vi "Log Text to Sinks.vi"(8 "error in (no error)":errorcluster, 10 "Log Text":string, 11 "Logger in":refnum<class "Logger.lvclass">) -> (0 "error out":errorcluster, 3 "Logger out":refnum<class "Logger.lvclass">)   [LabVIEW 2020, in "LV Logging.lvlib" / "Logger.lvclass"]
uses:
  Logger.lvclass
  Sink/Sink.lvclass
  LV Logging.lvlib
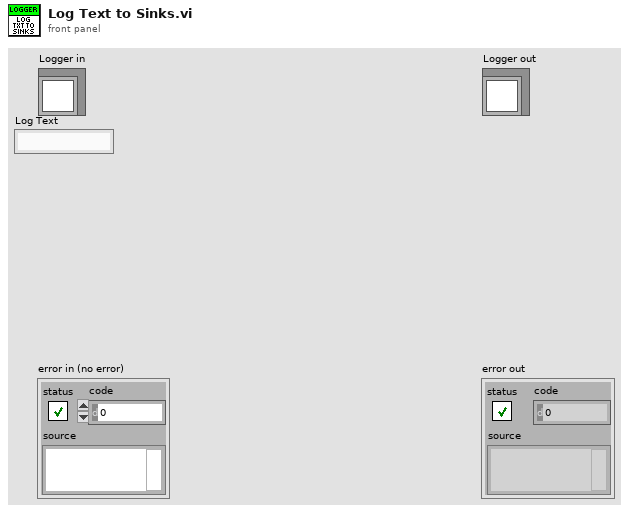
[diagram p1: front panel]
types:
  T1 = enum16{"Init", "Get Logger", "Register Sink", "Set Global Debug Level", "Get Sinks"}
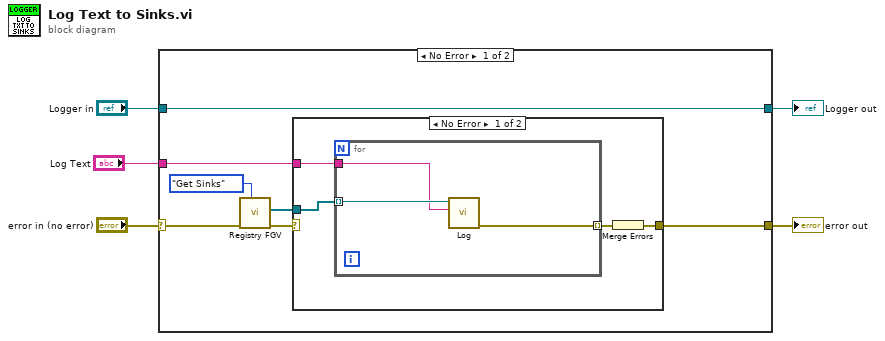
[diagram p0: block diagram]
diagram:
  n1 = case shown="No Error" "error in (no error)" {
    selector: "error in (no error)" -> [w11 w21]
    tunnel: [w6 w21] -> w4
    tunnel: [w12 w20] -> w2
    tunnel: "Logger in" -> [w12 w20]
    tunnel: "Log Text" -> [w7 _]
    frame No Error {
      n2 = call "Registry FGV.vi"("State (Get Logger)"=T1."Get Sinks", "error in (no error)"=w11) -> ("error out"=w9:errorcluster, "Sinks"=w8:refnum<class "Sink.lvclass">[])  [unwired: 6 in, 2 out]
      n3 = case shown="No Error" w9 {
        tunnel: w8 -> [w16 _]
        tunnel: w7 -> [w15 _]
        tunnel: [w13 _] -> w6
        frame No Error {
          n4 = for {
            tunnel: w16 -> [w19] mode=indexing
            tunnel: w15 -> [w18]
            tunnel: [w17] -> w14 mode=indexing
            n5 = call-dynamic "Log.vi"("Log Text"=w18, "Sink in"=w19) -> ("error out"=w17:errorcluster)  [unwired: 8 in, 1 out]
          }
          n6 = Merge Errors(w14) -> (w13:errorcluster)
        }
        frame Error {
        }
      }
    }
    frame Error {
    }
  }
  "error out" <- w4
  "Logger out" <- w2
